vi "niFpga wdp fft tf 128 U32 inv.vi"(4 "index":fxp<+,6,6>, 10 "enable":bool) -> (2 "imag":fxp<+/-,16,2>, 3 "real":fxp<+/-,16,2>)   [LabVIEW 2017]
uses:
  <vilib>/rvi/FXPMathLib/basic elements/FxpDiscreteDelay/XNode/nifxpmath_DiscreteDelay.xnode
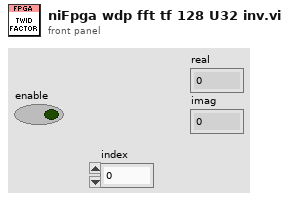
[diagram p1: front panel]
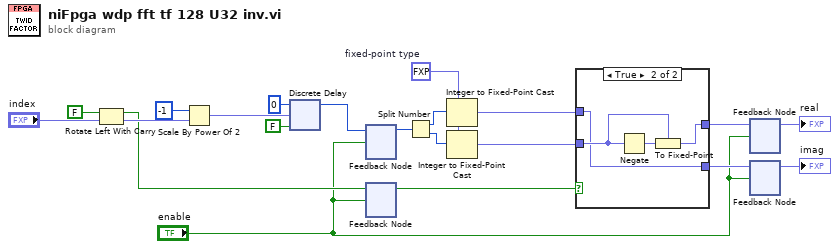
[diagram p0: block diagram]
diagram:
  w8 = fxp<+/-,16,2> 0.0  # fixed-point type
  n1 = Rotate Left With Carry(2:"index", 3:FALSE ("carry")) -> (0:w20:fxp<+,6,6>, 1:w12:bool)
  n2 = Scale By Power Of 2(n=i16 -1, x=w20) -> (x*2^n=w14:fxp<+,6,6>)
  n3 = xnode "Discrete Delay"("D"=u32 0, "n-1[0..31]"=w14, "enable"=FALSE) -> ("Q"=w13:u32)
  n4 = feedback-in #1(w13, "enable") -> ()
  n5 = feedback #1() -> (w17:u32)  [unwired: 1 in]
  n6 = feedback #2() -> (w11:bool)  [unwired: 1 in]
  n7 = feedback-in #2(w12, "enable") -> ()
  n8 = Split Number(x=w17) -> (hi(x)=w10:u16, lo(x)=w9:u16)
  n9 = Integer to Fixed-Point Cast(fixed-point type=w8, integer=w10) -> (fixed-point=w7:fxp<+/-,16,2>)
  n10 = Integer to Fixed-Point Cast(fixed-point type=w8, integer=w9) -> (fixed-point=w6:fxp<+/-,16,2>)
  n11 = case shown="True" w11 {
    tunnel: w7 -> [w23 w24]
    tunnel: w6 -> [w22 w26]
    tunnel: [w23 w25] -> w5
    tunnel: [w22 w24] -> w4
    frame False {
    }
    frame True {
      n12 = Negate(x=w26) -> (-x=w27:fxp<+/-,17,3>)
      n13 = To Fixed-Point(fixed-point type=w26, number=w27) -> (fixed-point=w25:fxp<+/-,16,2>)
    }
  }
  n14 = feedback #3() -> (→"real":fxp<+/-,16,2>)  [unwired: 1 in]
  n15 = feedback-in #3(w5, "enable") -> ()
  n16 = feedback #4() -> (→"imag":fxp<+/-,16,2>)  [unwired: 1 in]
  n17 = feedback-in #4(w4, "enable") -> ()
